vi "Shooter.vi"(0 "Encoder":dbl, 1 "4 Feet":bool, 2 "2 Feet":bool, 3 "Manual Shoot":bool) -> ()   [LabVIEW 2013]
panel:
  in  "4 Feet":dbl=200.0 format="%#_13g"
  in  "2 Feet":dbl=100.0 format="%#_13g"
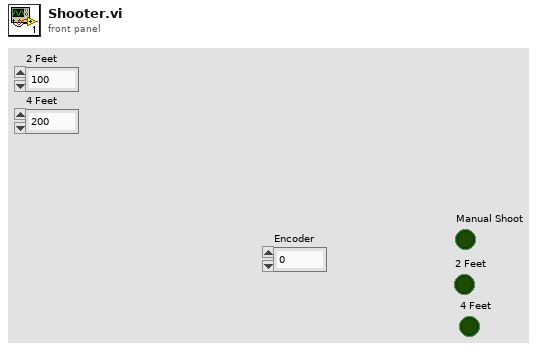
[diagram p1: front panel]
types:
  T1 = enum16{"No Shoot", "Manual Shoot", "2 Feet", "4 Feet"}
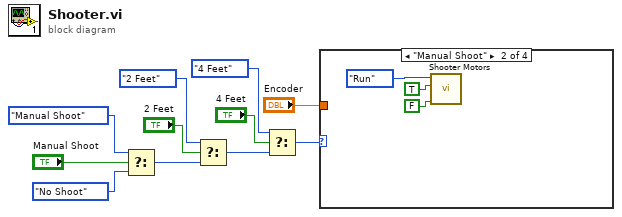
[diagram p0: block diagram]
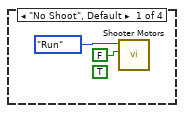
[diagram p2: hidden frame]
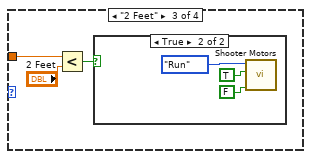
[diagram p3: hidden frame]
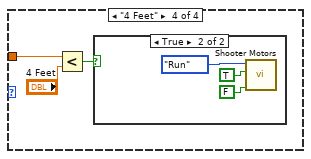
[diagram p5: hidden frame]
diagram:
  n1 = Select(t=T1."Manual Shoot" ("Shoot 2"), s="Manual Shoot", f=T1."No Shoot" ("Shoot 2")) -> (s? t:f=w7:T1)
  n2 = Select(t=T1."2 Feet" ("Shoot 2"), s="2 Feet", f=w7) -> (s? t:f=w4:T1)
  n3 = Select(t=T1."4 Feet" ("Shoot 2"), s="4 Feet", f=w4) -> (s? t:f=w2:T1)
  n4 = case shown="\"Manual Shoot\"" w2 {
    tunnel: "Encoder" -> [_ _ w18 w23]
    frame "No Shoot", Default {
      (unwired) TRUE ("Return")
      n5 = call "Shooter Motors.vi"("Fire"=FALSE, "State Control"=enum16{"Open", "Run", "End"}."Run") -> ()  [unwired: 2 in, 2 out]
    }
    frame "Manual Shoot" {
      n6 = call "Shooter Motors.vi"("Return"=FALSE, "Fire"=TRUE, "State Control"=enum16{"Open", "Run", "End"}."Run") -> ()  [unwired: 1 in, 2 out]
    }
    frame "2 Feet" {
      n7 = Less?(x=w18, y="2 Feet") -> (x < y?=w17:bool)
      n8 = case shown="True" w17 {
        frame False {
        }
        frame True {
          n9 = call "Shooter Motors.vi"("Return"=FALSE, "Fire"=TRUE, "State Control"=enum16{"Open", "Run", "End"}."Run") -> ()  [unwired: 1 in, 2 out]
        }
      }
    }
    frame "4 Feet" {
      n10 = Less?(x=w23, y="4 Feet") -> (x < y?=w24:bool)
      n11 = case shown="True" w24 {
        frame False {
        }
        frame True {
          n12 = call "Shooter Motors.vi"("Return"=FALSE, "Fire"=TRUE, "State Control"=enum16{"Open", "Run", "End"}."Run") -> ()  [unwired: 1 in, 2 out]
        }
      }
    }
  }
